vi "PH_SSAC.Frame Corrector.vi"(2 "Image Dimension":u32, 3 "Frame Dimension":u32) -> (0 "Corrected Frame Dimension":u32, 1 "Corrected Frame Start Point":u32)   [LabVIEW 2014, in "PH_SSAC.lvlib"]
doc: "This VI calculates the corrected values for the signal frames."
uses:
  PH_SSAC.lvlib
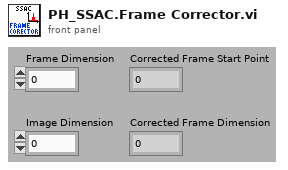
[diagram p1: front panel]
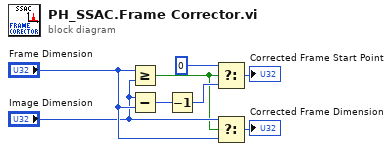
[diagram p0: block diagram]
diagram:
  n1 = Greater Or Equal?(x="Frame Dimension", y="Image Dimension") -> (x >= y?=w4:bool)
  n2 = Subtract(x="Image Dimension", y="Frame Dimension") -> (x-y=w3:u32)
  n3 = Decrement(x=w3) -> (x-1=w8:u32)
  n4 = Select(t=u32 0, s=w4, f=w8) -> (s? t:f=→"Corrected Frame Start Point":u32)
  n5 = Select(t="Image Dimension", s=w4, f="Frame Dimension") -> (s? t:f=→"Corrected Frame Dimension":u32)
